vi "prop_plot_main.vi"() -> ()   [LabVIEW 2020, in "3DPC_SurfacePlot.xctl"]
uses:
  <vilib>/Native 3D Graph/xcontrol/3DPC_SurfacePlot.xctl
  <vilib>/Native 3D Graph/typedefs/prop_plot_all_array.ctl
  <vilib>/Native 3D Graph/typedefs/prop_plot_all.ctl
  <vilib>/Native 3D Graph/typedefs/prop_plot_projection.ctl
  <vilib>/Native 3D Graph/typedefs/prop_plot_surface.ctl
  <vilib>/Native 3D Graph/typedefs/prop_plot_contour.ctl
  <vilib>/Native 3D Graph/typedefs/prop_plot_normal.ctl
  <vilib>/Native 3D Graph/typedefs/prop_plot_point_line.ctl
  <vilib>/Native 3D Graph/typedefs/range_cluster.ctl
  <vilib>/Native 3D Graph/typedefs/min_max.ctl
  <vilib>/Utility/miscctls.llb/LVPointTypeDef.ctl
  <vilib>/Utility/miscctls.llb/LVPositionTypeDef.ctl
  <vilib>/event_ctls.llb/eventvkey.ctl
panel:
  in  "add new":string="[add new]"
  in  "Min Max":T1
  in  "done":refnum<user-event>
  in  "quit":refnum<user-event>
  out "Plot Properties Out":T3
  in  "Plot Properties In":T3
  in  "Delete Plot":bool
  in  "Add Plot":bool
  in  "Plots":i32(listbox)
  in  "Tab Plot Prop":T10(tab)
  in  "Color Map Mode":u16(ring) items=["Absolute", "Relative"]
  in  "Autoscale":bool
  in  "Coordinate System":u16(ring) items=["Cartesian", "Cylindrical", "Spherical"]
  in  "Surface Opacity":dbl=1.0 caption="Opacity"
  in  "Surface Shading":bool
  in  "Surface Draw":bool
  in  "Color Ramp":dbl(ramp) caption="Color Map"
  in  "Point Size":sgl=1.0
  in  "PL Color":u32(colorbox) caption="Color"
  in  "PL Antialiasing":bool
  in  "Points/Lines":u16(ring) items=["None", "Points", "Lines", "Both"]
  in  "Point Style":u16(ring) items=["Point", "EmptySquare", "Asterisk", "Diamond", "EmptyCircle", "Circle", "X"]
  in  "Line Style":u16(ring) items=["Solid", "Dash", "Dot", "Dash Dot"]
  in  "Line Width":sgl=1.0
  in  "Level List":i32(listbox)
  in  "Mode":u16(ring) items=["Levels", "Intervals", "Level List"]
  in  "Anchored Num":dbl
  in  "Anchored at":bool
  in  "Levels":sgl
  in  "Contour Direction":u16(ring) caption="Axis" items=["X", "Y", "Z"]
  in  "Contour Width":dbl=1.0 caption="Width"
  in  "Contour Color":u32(colorbox) caption="Color"
  in  "Contour Antialiasing":bool
  in  "Contour Draw":bool
  in  "Contour Line Style":u16(ring) caption="Line Style" items=["Solid", "Dash", "Dot", "Dash Dot"]
  in  "Interval":sgl
  in  "Normal Color":u32(colorbox) caption="Color"
  in  "Normal Length":sgl=0.1 caption="Length"
  in  "Normal Width":sgl=3.0 caption="Width"
  in  "Normal Draw":bool
  in  "Normal Antialiasing":bool
  in  "Projection Draw XY":bool
  in  "Projection Draw YZ":bool
  in  "Projection Draw XZ":bool
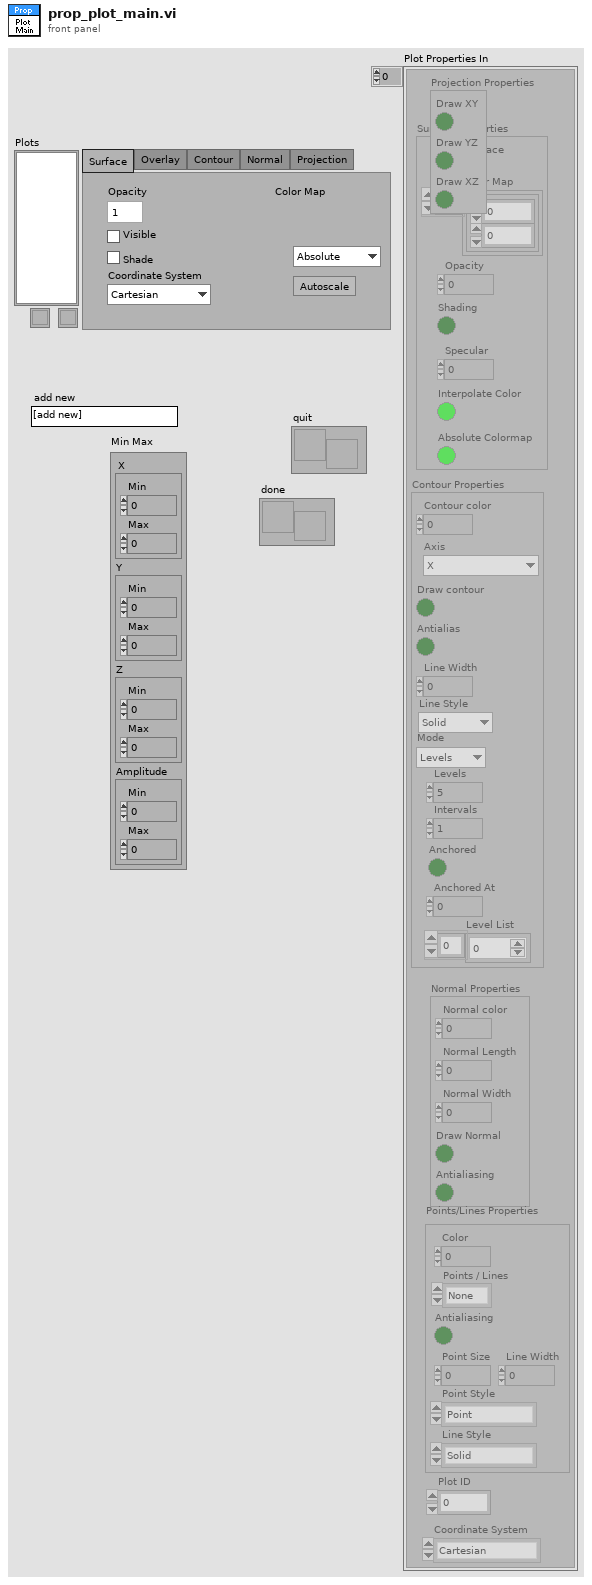
[diagram p1: front panel]
types:
  T1 = typedef "3DPC_SurfacePlot.xctl/range_cluster.ctl" = cluster{"X":T2, "Y":T2, "Z":T2, "Amplitude":T2}
  T2 = typedef "3DPC_SurfacePlot.xctl/min_max.ctl" = cluster{"Min":sgl, "Max":sgl}
  T3 = typedef "3DPC_SurfacePlot.xctl/prop_plot_all_array.ctl" = T4[]
  T4 = typedef "3DPC_SurfacePlot.xctl/prop_plot_all.ctl" = cluster{"Projection Properties":T5, "Surface Properties":T6, "Contour Properties":T7, "Normal Properties":T8, "Points/Lines Properties":T9, "Plot ID":i32, "Coordinate System":enum16{"Cartesian", "Cylindrical", "Spherical"}}
  T5 = typedef "3DPC_SurfacePlot.xctl/prop_plot_projection.ctl" = cluster{"Draw XY":bool, "Draw YZ":bool, "Draw XZ":bool}
  T6 = typedef "3DPC_SurfacePlot.xctl/prop_plot_surface.ctl" = cluster{"Draw surface":bool, "Opacity":dbl, "Shading":bool, "Specular":i32, "Color Map":cluster{dbl, u32}[], "Interpolate Color":bool, "Absolute Colormap":bool}
  T7 = typedef "3DPC_SurfacePlot.xctl/prop_plot_contour.ctl" = cluster{"Contour color":u32, "Axis":enum16{"X", "Y", "Z"}, "Draw contour":bool, "Antialias":bool, "Line Width":sgl, "Contour Line Style":enum16{"Solid", "Dash", "Dot", "Dash Dot"}, "Mode":enum16{"Levels", "Intervals", "Level List"}, "Levels":sgl, "Intervals":sgl, "Anchored At":sgl, "Anchored":bool, "Level List":dbl[]}
  T8 = typedef "3DPC_SurfacePlot.xctl/prop_plot_normal.ctl" = cluster{"Normal color":u32, "Normal Length":sgl, "Normal Width":sgl, "Draw Normal":bool, "Antialiasing":bool}
  T9 = typedef "3DPC_SurfacePlot.xctl/prop_plot_point_line.ctl" = cluster{"Color":u32, "Antialiasing":bool, "Point Size":sgl, "Points / Lines":enum16{"None", "Points", "Lines", "Both"}, "Point Style":enum16{"Point", "EmptySquare", "Asterisk", "Diamond", "EmptyCircle", "Circle", "X"}, "Line Style":enum16{"Solid", "Dash", "Dot", "Dash Dot"}, "Line Width":sgl}
  T10 = enum32{"Surface", "Overlay", "Contour", "Normal", "Projection"}
  T11 = typedef "LVPointTypeDef.ctl" = cluster{"Horizontal":i16, "Vertical":i16}
  T12 = typedef "LVPositionTypeDef.ctl" = cluster{"Left":i32, "Top":i32}
  T13 = typedef "eventvkey.ctl" = enum16{"ASCII", "Enter", "Return", "Shift", "Ctrl", "Alt", "Cmd", "Opt", "Caps", "NumLock", "Clear", "Break", "Up", "Down", "Left", "Right", "Insert", "Delete", "Home", "End", "PageUp", "PageDown", "Escape", "Help", "Pause", "ScrollLock", "F1", "F2", "F3", "F4", "F5", "F6", "F7", "F8", "F9", "F10", "F11", "F12", "F13", "F14", "F15", "F16", "F17", "F18", "F19", "F20", "F21", "F22", "F23", "F24", "Play", "VolumeUp", "VolumeDown", "Mute", "Two Byte Char"}
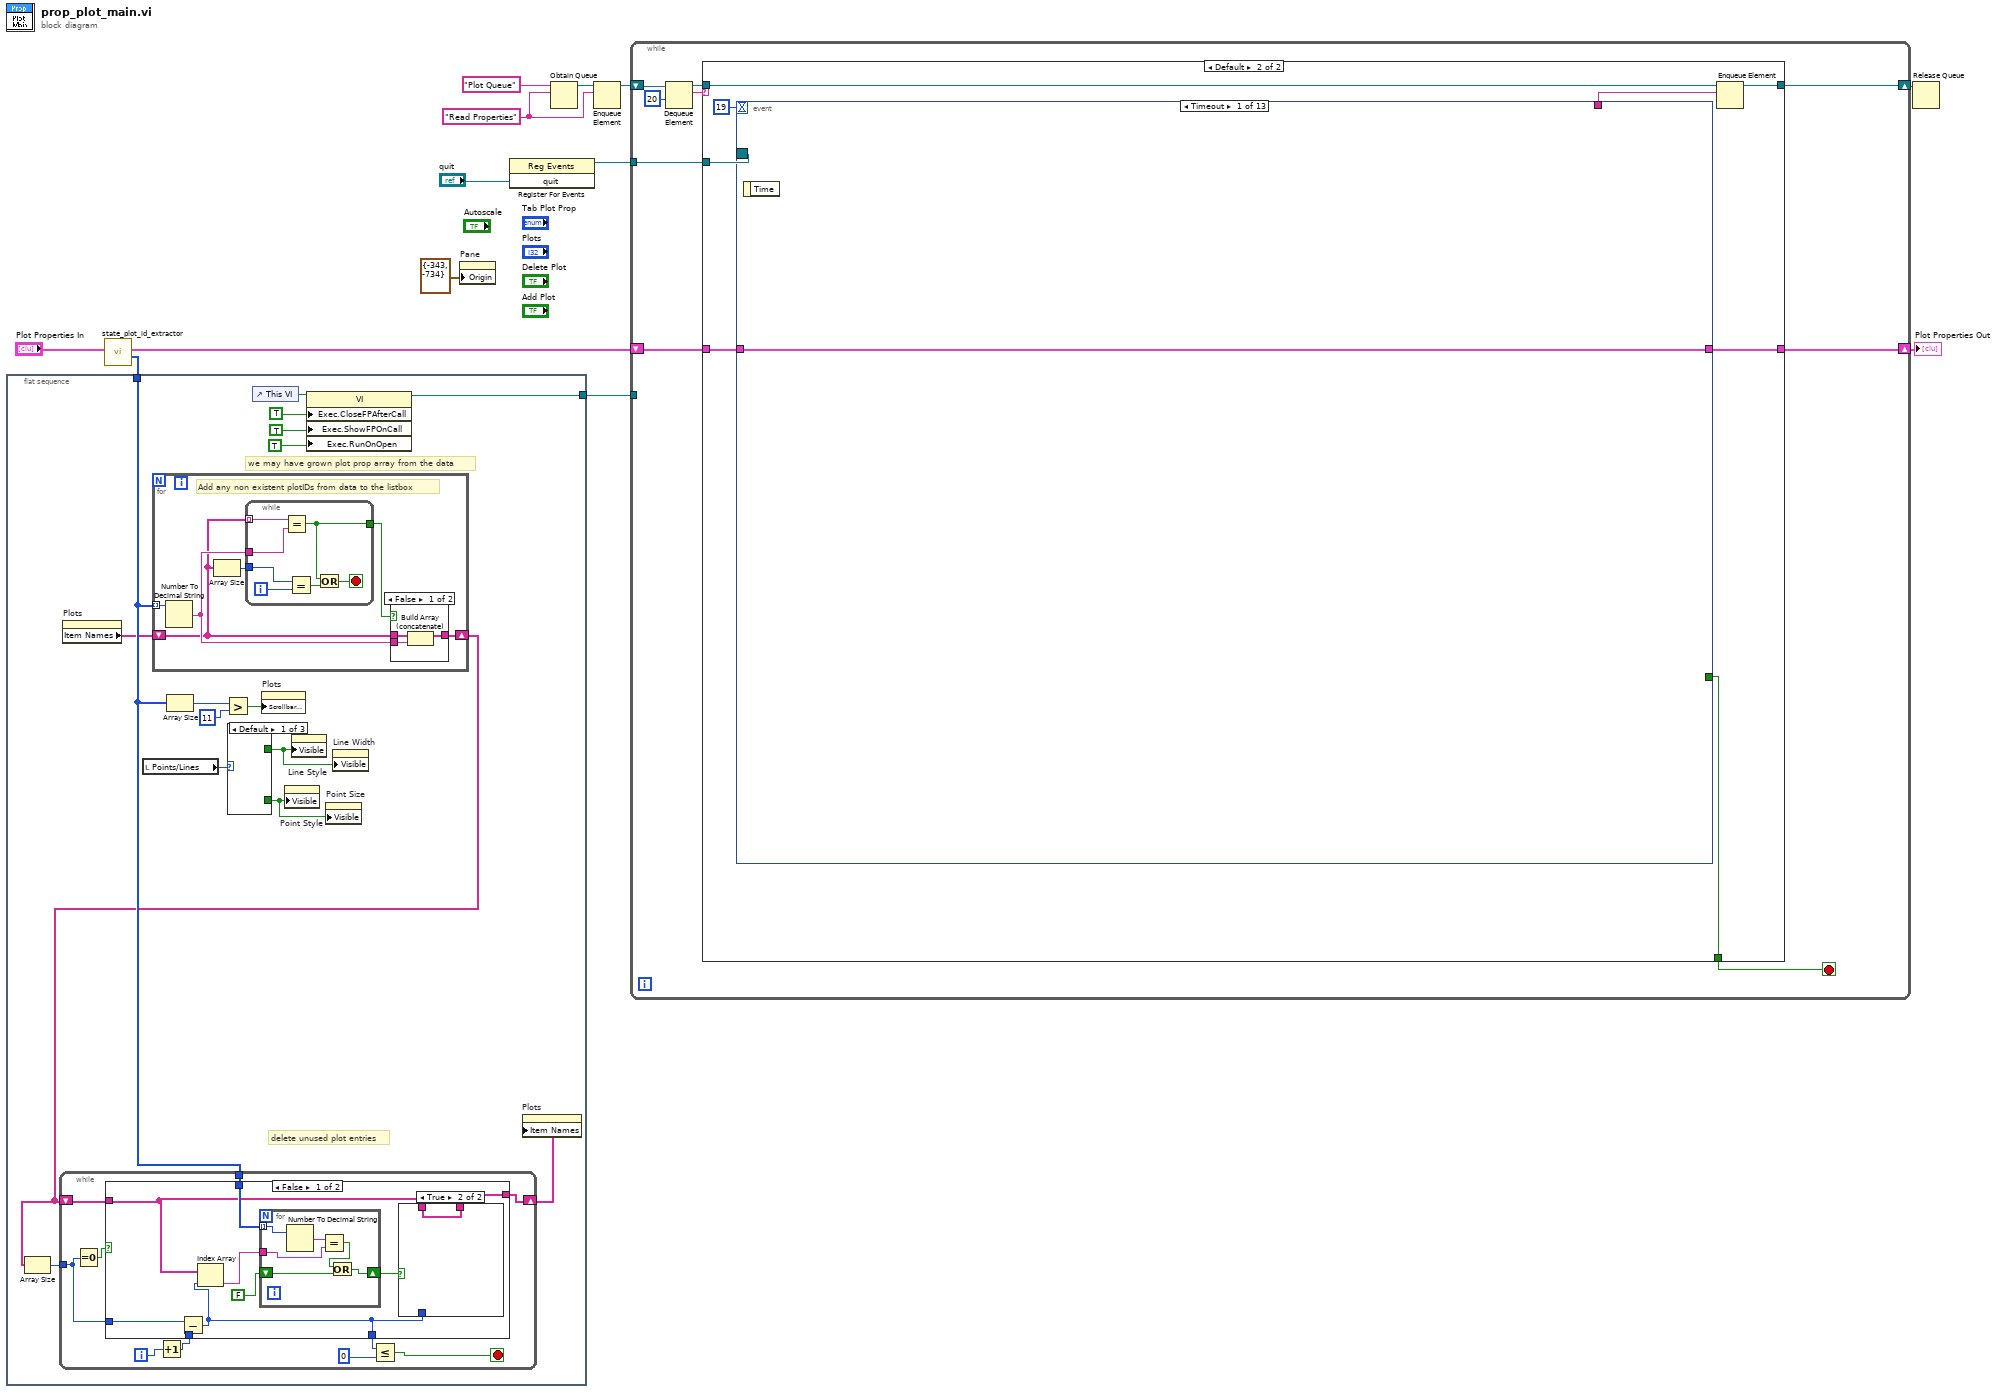
[diagram p0: block diagram]
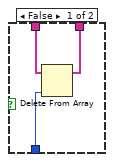
[diagram p2: hidden frame]
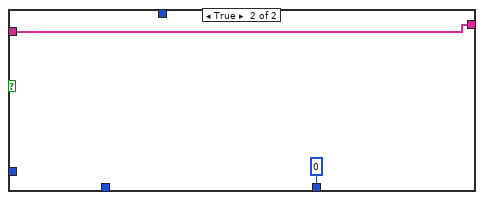
[diagram p3: hidden frame]
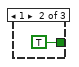
[diagram p4: hidden frame]
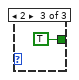
[diagram p5: hidden frame]
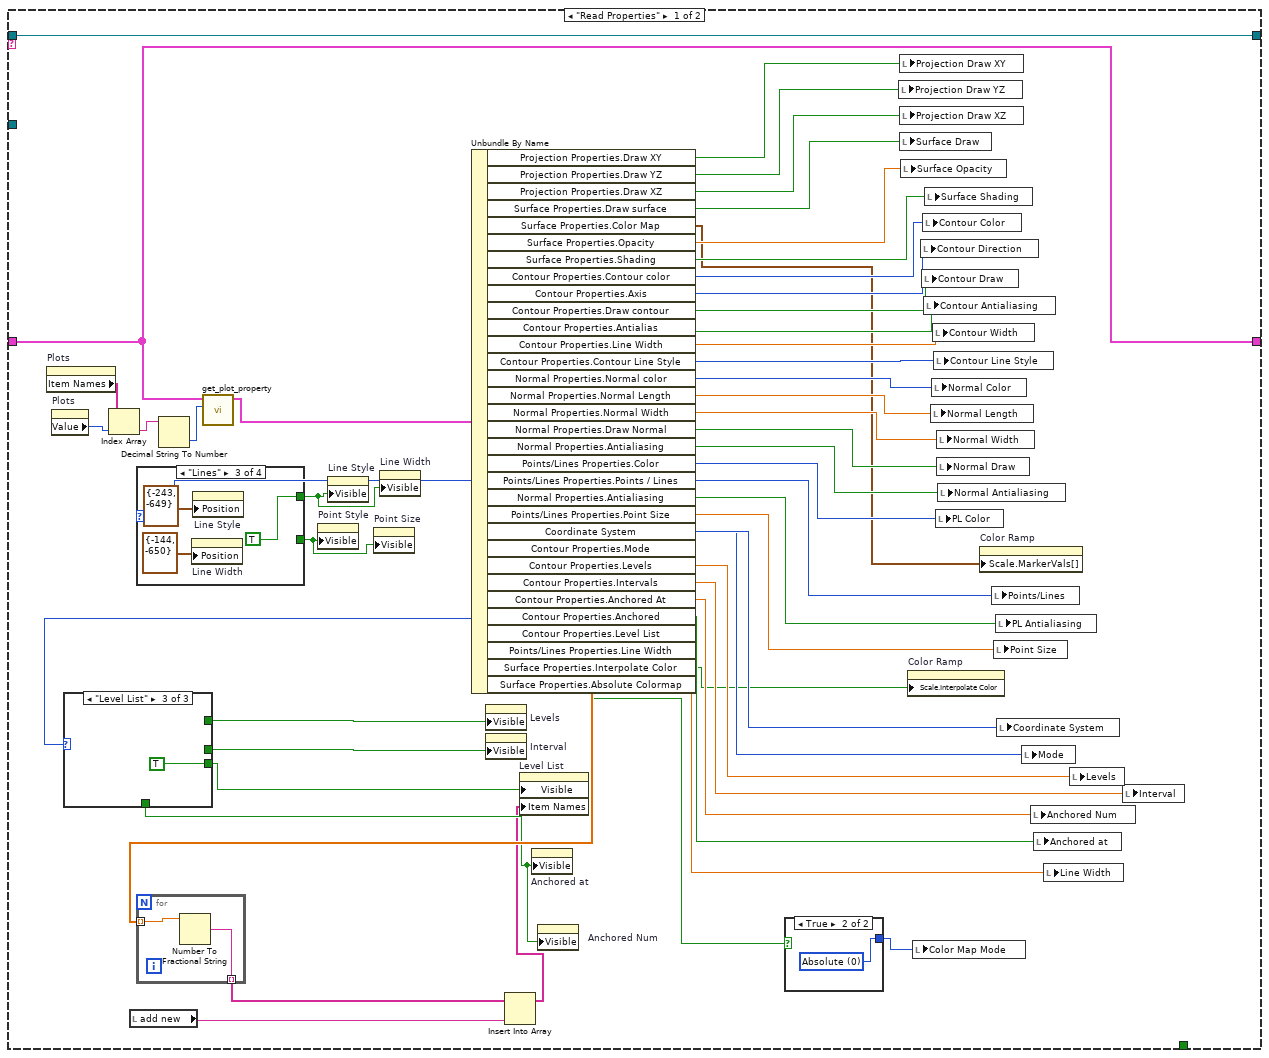
[diagram p7: hidden frame]
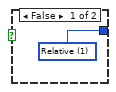
[diagram p8: hidden frame]
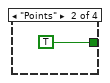
[diagram p10: hidden frame]
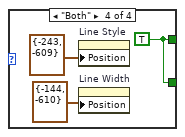
[diagram p11: hidden frame]
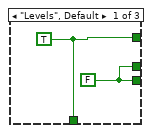
[diagram p12: hidden frame]
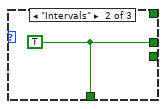
[diagram p13: hidden frame]
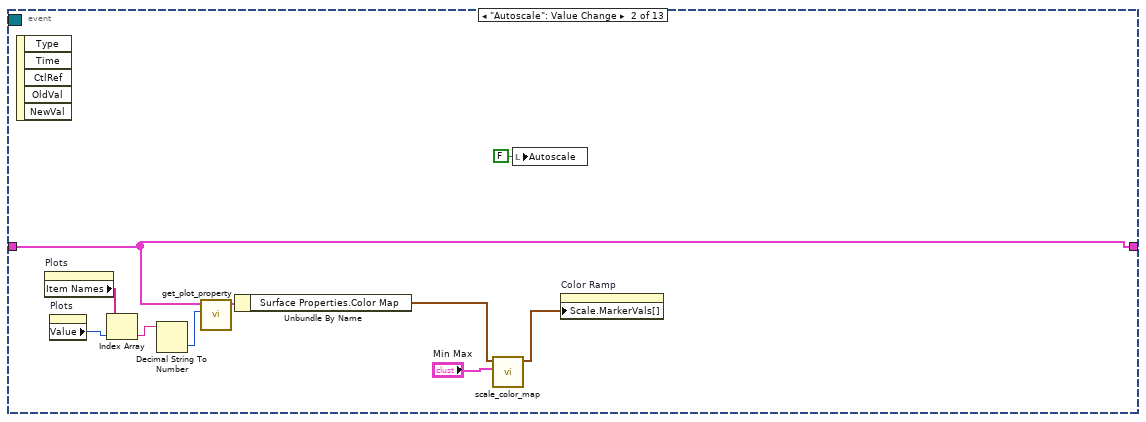
[diagram p14: hidden frame]
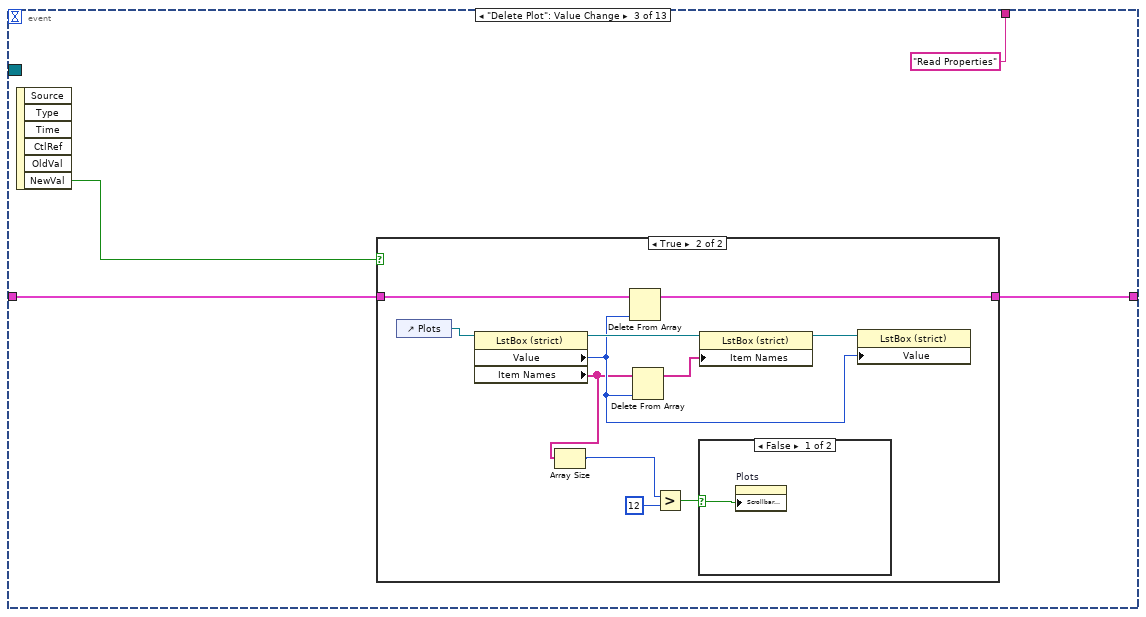
[diagram p15: hidden frame]
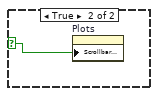
[diagram p17: hidden frame]
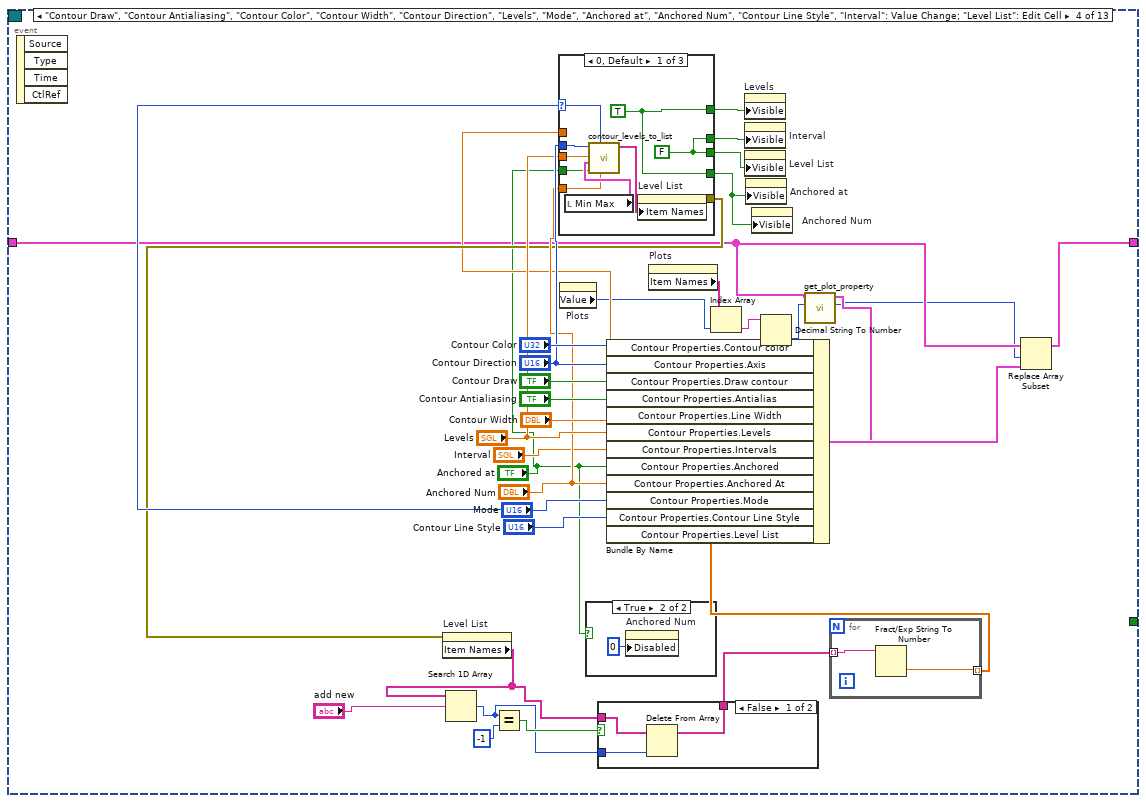
[diagram p18: hidden frame]
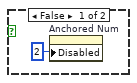
[diagram p19: hidden frame]
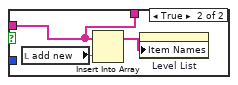
[diagram p20: hidden frame]
diagram:
  w11 = "Read Properties"
  n1 = flat-sequence {
    tunnel: [w29] -> w7
    tunnel: w4 -> [w28]
    frame #0 {
      # "delete unused plot entries"
      # "we may have grown plot prop array from the data"
      n2 = property on="Plots" class="LstBox (strict)"() -> ("Item Names"=w14:string[])  [unwired: 2 in, 2 out]
      n3 = local read "Points/Lines"() -> (w21:u16)
      n4 = for {
        tunnel: w28 -> [w66] mode=indexing
        shift-right: [w64] -> w16
        shift-left: w14 -> [w63]
        # "Add any non existent plotIDs from data to the listbox"
        n5 = Number To Decimal String(number=w66) -> (decimal integer string=w65:string)  [unwired: 1 out]
        n6 = Array Size(array=w63) -> (size(s)=w68:i32)
        n7 = while {
          tunnel: w63 -> [w79] mode=indexing
          tunnel: w68 -> [w78]
          tunnel: [w74] -> w67
          tunnel: w65 -> [w73]
          i -> [w77]
          stop <- w75 stop-if-true
          n8 = Equal?(x=w79, y=w73) -> (x = y?=w74:bool)
          n9 = Equal?(x=w78, y=w77) -> (x = y?=w76:bool)
          n10 = Or(x=w74, y=w76) -> (x .or. y?=w75:bool)
        }
        n11 = case shown="False" w67 {
          tunnel: w65 -> [w71 _]
          tunnel: [w70 w72] -> w64
          tunnel: w63 -> [w69 w72]
          frame False {
            n12 = Build Array (concatenate)(w69, w71) -> (w70:string[])
          }
          frame True {
          }
        }
      }
      n13 = Array Size(array=w16) -> (size(s)=w15:i32)
      n14 = while {
        tunnel: w28 -> [w37]
        shift-right: [w36] -> w17
        shift-left: w16 -> [w35]
        tunnel: w15 -> [w31]
        i -> [w38]
        stop <- w32 stop-if-true
        n15 = Equal To 0?(x=w31) -> (x = 0?=w30:bool)
        n16 = Increment(x=w38) -> (x+1=w39:i32)
        n17 = case shown="False" w30 {
          tunnel: w39 -> [w48 _]
          tunnel: w37 -> [w47 _]
          tunnel: [w44 w60] -> w36
          tunnel: w35 -> [w42 w60]
          tunnel: [w41 0] -> w34
          tunnel: w31 -> [w40 _]
          frame False {
            n18 = Subtract(x=w40, y=w48) -> (x-y=w41:i32)
            n19 = Index Array(array=w42, index=w41) -> (element=w46:string)
            n20 = for {
              tunnel: w47 -> [w58] mode=indexing
              tunnel: w46 -> [w56]
              shift-right: [w53] -> w43
              shift-left: FALSE -> [w55]
              n21 = Number To Decimal String(number=w58) -> (decimal integer string=w57:string)  [unwired: 1 out]
              n22 = Equal?(x=w57, y=w56) -> (x = y?=w54:bool)
              n23 = Or(x=w54, y=w55) -> (x .or. y?=w53:bool)
            }
            n24 = case shown="True" w43 {
              tunnel: w42 -> [w50 w52]
              tunnel: w41 -> [w51 _]
              tunnel: [w49 w52] -> w44
              frame False {
                n25 = Delete From Array(array=w50, index=w51) -> (array with subset deleted=w49:string[])  [unwired: 1 in, 1 out]
              }
              frame True {
              }
            }
          }
          frame True {
          }
        }
        n26 = Less Or Equal?(x=w34, y=0) -> (x <= y?=w32:bool)
      }
      n27 = Array Size(array=w28) -> (size(s)=w20:i32)
      n28 = Greater?(x=w20, y=11) -> (0:w18:bool)
      n29 = case shown="Default" w21 {
        tunnel: [_ TRUE ("Visible") _] -> w23
        tunnel: [_ _ TRUE ("Visible")] -> w22
        frame Default {
        }
        frame 1 {
        }
        frame 2 {
        }
      }
      n30 = control-ref of="This VI"() -> (w27:refnum<vi>)
      n31 = property on="Plots" class="LstBox (strict)"("Scrollbar Visible"=w18) -> ()  [unwired: 2 in, 2 out]
      n32 = property on="Point Style" class="Ring (strict)"("Visible"=w23) -> ()  [unwired: 2 in, 2 out]
      n33 = property on="Line Style" class="Ring (strict)"("Visible"=w22) -> ()  [unwired: 2 in, 2 out]
      n34 = property class="VI"(reference=w27, "Exec.CloseFPAfterCall"=TRUE ("Execution:Close After Call"), "Exec.ShowFPOnCall"=TRUE ("Execution:Show Front Panel On Call"), "Exec.RunOnOpen"=TRUE ("Execution:Run When Opened")) -> (reference out=w29:refnum<vi>)  [unwired: 1 in, 1 out]
      n35 = property on="Point Size" class="DigNum (strict)"("Visible"=w23) -> ()  [unwired: 2 in, 2 out]
      n36 = property on="Line Width" class="DigNum (strict)"("Visible"=w22) -> ()  [unwired: 2 in, 2 out]
      n37 = property on="Plots" class="LstBox (strict)"("Item Names"=w17) -> ()  [unwired: 2 in, 2 out]
    }
  }
  n38 = call <vilib>:"state_plot_id_extractor.vi"("Plot Properties Array In"="Plot Properties In") -> ("Plot IDs"=w4:i32[], "Plot Properties Array Out"=w5:T3)  [unwired: 9 out]
  n39 = property on="Pane" class="Pane"("Origin"=T11 {"Horizontal"=-343, "Vertical"=-734} ("Point")) -> ()  [unwired: 2 in, 2 out]
  n40 = register-events("quit") -> (reference out=w2:refnum<event-registration>)  [unwired: 2 in, 1 out]
  n41 = Obtain Queue(name (unnamed)="Plot Queue", element data type=w11) -> (queue out=w12:refnum<queue>)  [unwired: 3 in, 2 out]
  n42 = Enqueue Element(queue=w12, element=w11) -> (queue out=w10:refnum<queue>)  [unwired: 1 in, 3 out]
  n43 = while {
    shift-right: [w87] -> w9
    shift-left: w5 -> [w88]
    shift-right: [w82] -> w8
    shift-left: w10 -> [w85]
    tunnel: w7 -> [_]
    tunnel: w2 -> [w81]
    stop <- w80 stop-if-true
    n44 = Dequeue Element(queue=w85, timeout in ms (-1)=20) -> (queue out=w83:refnum<queue>, element=w84:string)  [unwired: 1 in, 2 out]
    n45 = case shown="Default" w84 {
      tunnel: w88 -> [w98 w157]
      tunnel: [w98 w156] -> w87
      tunnel: w83 -> [w137 w160]
      tunnel: [w137 w159] -> w82
      tunnel: w81 -> [_ w154]
      tunnel: [_ w153] -> w80
      frame "Read Properties" {
        n46 = property on="Plots" class="LstBox (strict)"() -> ("Item Names"=w96:string[])  [unwired: 2 in, 2 out]
        n47 = property on="Plots" class="LstBox (strict)"() -> ("Value"=w95:i32)  [unwired: 2 in, 2 out]
        n48 = Index Array(array=w96, index=w95) -> (element=w94:string)
        n49 = local read "add new"() -> (w99:string)
        n50 = Decimal String To Number(string=w94) -> (number=w93:i32)  [unwired: 3 out]
        n51 = call <vilib>:"get_plot_property.vi"("Plot ID"=w93, "Plot Properties Array"=w98) -> ("element"=w97:T4)  [unwired: 1 in, 8 out]
        n52 = Unbundle By Name(w97) -> ("Projection Properties.Draw XY"=w136:bool, "Projection Properties.Draw YZ"=w135:bool, "Projection Properties.Draw XZ"=w134:bool, "Surface Properties.Draw surface"=w133:bool, "Surface Properties.Color Map"=w92:cluster{dbl, u32}[], "Surface Properties.Opacity"=w132:dbl, "Surface Properties.Shading"=w131:bool, "Contour Properties.Contour color"=w130:u32, "Contour Properties.Axis"=w129:enum16{"X", "Y", "Z"}, "Contour Properties.Draw contour"=w128:bool, "Contour Properties.Antialias"=w127:bool, "Contour Properties.Line Width"=w126:sgl, "Contour Properties.Contour Line Style"=w116:enum16{"Solid", "Dash", "Dot", "Dash Dot"}, "Normal Properties.Normal color"=w125:u32, "Normal Properties.Normal Length"=w124:sgl, "Normal Properties.Normal Width"=w123:sgl, "Normal Properties.Draw Normal"=w122:bool, "Normal Properties.Antialiasing"=w121:bool, "Points/Lines Properties.Color"=w120:u32, "Points/Lines Properties.Points / Lines"=w101:enum16{"None", "Points", "Lines", "Both"}, "Normal Properties.Antialiasing"=w119:bool, "Points/Lines Properties.Point Size"=w118:sgl, "Coordinate System"=w117:enum16{"Cartesian", "Cylindrical", "Spherical"}, "Contour Properties.Mode"=w113:enum16{"Levels", "Intervals", "Level List"}, "Contour Properties.Levels"=w111:sgl, "Contour Properties.Intervals"=w110:sgl, "Contour Properties.Anchored At"=w109:sgl, "Contour Properties.Anchored"=w108:bool, "Contour Properties.Level List"=w107:dbl[], "Points/Lines Properties.Line Width"=w100:sgl, "Surface Properties.Interpolate Color"=w91:bool, "Surface Properties.Absolute Colormap"=w90:bool)
        n53 = case shown="\"Level List\"" w113 {
          tunnel: [w149 _ _] -> w115
          tunnel: [w150 w151 _] -> w114
          tunnel: [w150 _ TRUE ("Visible")] -> w112
          tunnel: [w149 w151 _] -> w106
          frame "Levels", Default {
            w150 = FALSE ("Visible")
            w149 = TRUE ("Visible")
          }
          frame "Intervals" {
            w151 = TRUE ("Visible")
          }
          frame "Level List" {
          }
        }
        n54 = case shown="\"Lines\"" w101 {
          tunnel: [_ TRUE ("Visible") _ w144] -> w102
          tunnel: [_ _ TRUE ("Visible") w144] -> w103
          frame "None", Default {
          }
          frame "Points" {
          }
          frame "Lines" {
            n55 = property on="Line Width" class="DigNum (strict)"("Position"=T12 {"Left"=-144, "Top"=-650} ("Position 3")) -> ()  [unwired: 2 in, 2 out]
            n56 = property on="Line Style" class="Ring (strict)"("Position"=T12 {"Left"=-243, "Top"=-649} ("Position 2")) -> ()  [unwired: 2 in, 2 out]
          }
          frame "Both" {
            w144 = TRUE ("Visible")
            n57 = property on="Line Style" class="Ring (strict)"("Position"=T12 {"Left"=-243, "Top"=-609} ("Position 4")) -> ()  [unwired: 2 in, 2 out]
            n58 = property on="Line Width" class="DigNum (strict)"("Position"=T12 {"Left"=-144, "Top"=-610} ("Position 5")) -> ()  [unwired: 2 in, 2 out]
          }
        }
        n59 = for {
          tunnel: w107 -> [w148] mode=indexing
          tunnel: [w147] -> w105 mode=indexing
          n60 = Number To Fractional String(number=w148) -> (F-format string=w147:string)  [unwired: 3 out]
        }
        n61 = property on="Point Style" class="Ring (strict)"("Visible"=w102) -> ()  [unwired: 2 in, 2 out]
        n62 = property on="Line Style" class="Ring (strict)"("Visible"=w103) -> ()  [unwired: 2 in, 2 out]
        n63 = property on="Point Size" class="DigNum (strict)"("Visible"=w102) -> ()  [unwired: 2 in, 2 out]
        n64 = property on="Line Width" class="DigNum (strict)"("Visible"=w103) -> ()  [unwired: 2 in, 2 out]
        n65 = property on="Levels" class="DigNum (strict)"("Visible"=w115) -> ()  [unwired: 2 in, 2 out]
        n66 = property on="Interval" class="DigNum (strict)"("Visible"=w114) -> ()  [unwired: 2 in, 2 out]
        n67 = Insert Into Array(array=w105, new element=w99) -> (w104:string[])  [unwired: 1 in]
        n68 = property on="Level List" class="LstBox (strict)"("Visible"=w112, "Item Names"=w104) -> ()  [unwired: 2 in, 2 out]
        n69 = property on="Anchored at" class="Bool (strict)"("Visible"=w106) -> ()  [unwired: 2 in, 2 out]
        n70 = property on="Anchored Num" class="DigNum (strict)"("Visible"=w106) -> ()  [unwired: 2 in, 2 out]
        n71 = case shown="True" w90 {
          tunnel: [w138 w139] -> w89
          frame False {
            w138 = u16 1 items=["Absolute", "Relative"] ("Color Map Mode")
          }
          frame True {
            w139 = u16 0 items=["Absolute", "Relative"] ("Color Map Mode")
          }
        }
        n72 = local write "Projection Draw YZ"(w135) -> ()
        n73 = local write "Projection Draw XY"(w136) -> ()
        n74 = local write "Projection Draw XZ"(w134) -> ()
        n75 = local write "Surface Draw"(w133) -> ()
        n76 = local write "Surface Opacity"(w132) -> ()
        n77 = property on="Color Ramp" class="ColRmp (strict)"("Scale.Interpolate Color"=w91) -> ()  [unwired: 2 in, 2 out]
        n78 = local write "Color Map Mode"(w89) -> ()
        n79 = local write "Contour Direction"(w129) -> ()
        n80 = local write "Contour Draw"(w128) -> ()
        n81 = local write "Contour Color"(w130) -> ()
        n82 = local write "Contour Antialiasing"(w127) -> ()
        n83 = local write "Surface Shading"(w131) -> ()
        n84 = local write "Normal Length"(w124) -> ()
        n85 = local write "Normal Color"(w125) -> ()
        n86 = local write "Contour Width"(w126) -> ()
        n87 = local write "Contour Line Style"(w116) -> ()
        n88 = local write "PL Color"(w120) -> ()
        n89 = local write "Normal Width"(w123) -> ()
        n90 = local write "Normal Draw"(w122) -> ()
        n91 = local write "Normal Antialiasing"(w121) -> ()
        n92 = property on="Color Ramp" class="ColRmp (strict)"("Scale.MarkerVals[]"=w92) -> ()  [unwired: 2 in, 2 out]
        n93 = local write "Points/Lines"(w101) -> ()
        n94 = local write "Point Size"(w118) -> ()
        n95 = local write "PL Antialiasing"(w119) -> ()
        n96 = local write "Coordinate System"(w117) -> ()
        n97 = local write "Mode"(w113) -> ()
        n98 = local write "Anchored Num"(w109) -> ()
        n99 = local write "Anchored at"(w108) -> ()
        n100 = local write "Line Width"(w100) -> ()
        n101 = local write "Levels"(w111) -> ()
        n102 = local write "Interval"(w110) -> ()
      }
      frame Default {
        n103 = event shown="[0] Timeout" {
          selector: w154 -> [_ _ _ _ _ _ _ _ _ _ _ _ _]
          dyn-events: _ -> [_ _ _ _ _ _ _ _ _ _ _ _ _]
          timeout: 19 -> [_ _ _ _ _ _ _ _ _ _ _ _ _]
          tunnel: [_ _ "Read Properties" ("element") _ _ _ "Read Properties" ("element") _ _ "Read Properties" ("element") _ _ _] -> w158
          tunnel: w157 -> [w161 w166 w174 w194 w252 w289 w302 w312 w322 w339 w357 w368 w401]
          tunnel: [w161 w166 w173 w220 w251 w298 w308 w319 w329 w338 w362 w383 w415] -> w156
          tunnel: [_ _ _ _ _ _ _ _ TRUE _ _ _ _] -> w153
          event Timeout {
            n104 = event-data() -> ()  [unwired: 2 out]
          }
          event "Autoscale": Value Change {
            n105 = event-data() -> ()  [unwired: 6 out]
            n106 = property on="Plots" class="LstBox (strict)"() -> ("Item Names"=w171:string[])  [unwired: 2 in, 2 out]
            n107 = property on="Plots" class="LstBox (strict)"() -> ("Value"=w170:i32)  [unwired: 2 in, 2 out]
            n108 = Index Array(array=w171, index=w170) -> (element=w169:string)
            n109 = Decimal String To Number(string=w169) -> (number=w168:i32)  [unwired: 3 out]
            n110 = call <vilib>:"get_plot_property.vi"("Plot ID"=w168, "Plot Properties Array"=w166) -> ("element"=w167:T4)  [unwired: 1 in, 8 out]
            n111 = Unbundle By Name(w167) -> ("Surface Properties.Color Map"=w164:cluster{dbl, u32}[])
            n112 = call <vilib>:"scale_color_map.vi"("Min Max"="Min Max", "Color Map In"=w164) -> ("Color Map Out"=w163:cluster{dbl, u32}[])  [unwired: 9 out]
            n113 = local write "Autoscale"(FALSE ("Autoscale")) -> ()
            n114 = property on="Color Ramp" class="ColRmp (strict)"("Scale.MarkerVals[]"=w163) -> ()  [unwired: 2 in, 2 out]
          }
          event "Delete Plot": Value Change {
            n115 = event-data() -> ("NewVal"=w175:bool)  [unwired: 6 out]
            n116 = case shown="True" w175 {
              tunnel: w174 -> [w176 w187]
              tunnel: [w176 w186] -> w173
              frame False {
              }
              frame True {
                n117 = control-ref of="Plots"() -> (w184:refnum<vi>)
                n118 = property on="Property Node" class="LstBox (strict)"(reference=w184) -> (reference out=w183:refnum<vi>, "Value"=w181:i32, "Item Names"=w178:string[])  [unwired: 1 in, 1 out]
                n119 = Array Size(array=w178) -> (size(s)=w177:i32)
                n120 = Delete From Array(array=w187, index=w181) -> (array with subset deleted=w186:T3)  [unwired: 1 in, 1 out]
                n121 = Delete From Array(array=w178, index=w181) -> (array with subset deleted=w185:string[])  [unwired: 1 in, 1 out]
                n122 = Greater?(x=w177, y=12) -> (0:w180:bool)
                n123 = case shown="False" w180 {
                  selector: w180 -> [w188 w189]
                  frame False {
                    n124 = property on="Plots" class="LstBox (strict)"("Scrollbar Visible"=w188) -> ()  [unwired: 2 in, 2 out]
                  }
                  frame True {
                    n125 = property on="Plots" class="LstBox (strict)"("Scrollbar Visible"=w189) -> ()  [unwired: 2 in, 2 out]
                  }
                }
                n126 = property on="Property Node" class="LstBox (strict)"(reference=w183, "Item Names"=w185) -> (reference out=w182:refnum<vi>)  [unwired: 1 in, 1 out]
                n127 = property class="LstBox (strict)"(reference=w182, "Value"=w181) -> ()  [unwired: 1 in, 2 out]
              }
            }
          }
          event "Contour Draw", "Contour Antialiasing", "Contour Color", "Contour Width", "Contour Direction", "Levels", "Mode", "Anchored at", "Anchored Num", "Contour Line Style", "Interval": Value Change; "Level List": Edit Cell {
            n128 = event-data() -> ()  [unwired: 5 out]
            n129 = case shown="0, Default" "Mode" {
              selector: "Mode" -> [w230 w242 _]
              tunnel: [w238 _ _] -> w212
              tunnel: [w239 w247 _] -> w211
              tunnel: [w239 _ TRUE ("Visible")] -> w210
              tunnel: [w238 w247 _] -> w209
              tunnel: "Contour Direction" -> [w237 w243 _]
              tunnel: "Levels" -> [w231 _ _]
              tunnel: "Anchored at" -> [w235 w244 _]
              tunnel: "Anchored Num" -> [w234 w241 _]
              tunnel: [w232 _ _] -> w205
              tunnel: "Interval" -> [_ w240 _]
              frame 0, Default {
                w239 = FALSE ("Visible")
                w238 = TRUE ("Visible")
                n130 = local read "Min Max"() -> (w236:T1)
                n131 = call <vilib>:"contour_levels_to_list.vi"("Anchored Num"=w234, "Mode"=w230, "Anchored at"=w235, "Min Max"=w236, "Levels/Int"=w231, "Dimension"=w237) -> ("Item Names"=w233:string[])  [unwired: 5 out]
                n132 = property on="Level List" class="LstBox (strict)"("Item Names"=w233) -> (error out=w232:errorcluster)  [unwired: 2 in, 1 out]
              }
              frame 1 {
                w247 = TRUE ("Visible")
                n133 = local read "Min Max"() -> (w245:T1)
                n134 = call <vilib>:"contour_levels_to_list.vi"("Anchored Num"=w241, "Mode"=w242, "Anchored at"=w244, "Min Max"=w245, "Levels/Int"=w240, "Dimension"=w243) -> ("Item Names"=w246:string[])  [unwired: 5 out]
                n135 = property on="Level List" class="LstBox (strict)"("Item Names"=w246) -> ()  [unwired: 2 in, 2 out]
              }
              frame 2 {
              }
            }
            n136 = property on="Level List" class="LstBox (strict)"(error in=w205) -> ("Item Names"=w201:string[])  [unwired: 1 in, 2 out]
            n137 = Search 1D Array(1D array=w201, element="add new") -> (index of element=w200:i32)  [unwired: 1 out]
            n138 = Equal?(x=w200, y=-1) -> (x = y?=w202:bool)
            n139 = property on="Plots" class="LstBox (strict)"() -> ("Value"=w192:i32)  [unwired: 2 in, 2 out]
            n140 = case shown="True" "Anchored at" {
              frame False {
                n141 = property on="Anchored Num" class="DigNum (strict)"("Disabled"=u8 2) -> ()  [unwired: 2 in, 2 out]
              }
              frame True {
                n142 = property on="Anchored Num" class="DigNum (strict)"("Disabled"=u8 0) -> ()  [unwired: 2 in, 2 out]
              }
            }
            n143 = case shown="False" w202 {
              tunnel: w201 -> [w224 w229]
              tunnel: [w225 w229] -> w199
              tunnel: w200 -> [w226 _]
              frame False {
                n144 = Delete From Array(array=w224, index=w226) -> (array with subset deleted=w225:string[])  [unwired: 1 in, 1 out]
              }
              frame True {
                n145 = local read "add new"() -> (w227:string)
                n146 = Insert Into Array(array=w229, new element=w227) -> (w228:string[])  [unwired: 1 in]
                n147 = property on="Level List" class="LstBox (strict)"("Item Names"=w228) -> ()  [unwired: 2 in, 2 out]
              }
            }
            n148 = property on="Plots" class="LstBox (strict)"() -> ("Item Names"=w196:string[])  [unwired: 2 in, 2 out]
            n149 = Index Array(array=w196, index=w192) -> (element=w195:string)
            n150 = property on="Levels" class="DigNum (strict)"("Visible"=w212) -> ()  [unwired: 2 in, 2 out]
            n151 = property on="Interval" class="DigNum (strict)"("Visible"=w211) -> ()  [unwired: 2 in, 2 out]
            n152 = property on="Level List" class="LstBox (strict)"("Visible"=w210) -> ()  [unwired: 2 in, 2 out]
            n153 = property on="Anchored at" class="Bool (strict)"("Visible"=w209) -> ()  [unwired: 2 in, 2 out]
            n154 = property on="Anchored Num" class="DigNum (strict)"("Visible"=w209) -> ()  [unwired: 2 in, 2 out]
            n155 = Decimal String To Number(string=w195) -> (number=w191:i32)  [unwired: 3 out]
            n156 = call <vilib>:"get_plot_property.vi"("Plot ID"=w191, "Plot Properties Array"=w194) -> ("index of element"=w190:i32, "element"=w193:T4)  [unwired: 1 in, 7 out]
            n157 = for {
              tunnel: w199 -> [w250] mode=indexing
              tunnel: [w249] -> w214 mode=indexing
              n158 = Fract/Exp String To Number(string=w250) -> (number=w249:dbl)  [unwired: 4 out]
            }
            n159 = Bundle By Name(cluster=w193, "Contour Properties.Contour color"="Contour Color", "Contour Properties.Axis"="Contour Direction", "Contour Properties.Draw contour"="Contour Draw", "Contour Properties.Antialias"="Contour Antialiasing", "Contour Properties.Line Width"="Contour Width", "Contour Properties.Levels"="Levels", "Contour Properties.Intervals"="Interval", "Contour Properties.Anchored"="Anchored at", "Contour Properties.Anchored At"="Anchored Num", "Contour Properties.Mode"="Mode", "Contour Properties.Contour Line Style"="Contour Line Style", "Contour Properties.Level List"=w214) -> (w221:T4)
            n160 = Replace Array Subset(array=w194, new element=w221, index=w190) -> (w220:T3)
          }
          event "Level List": Key Down {
            n161 = event-data() -> ("VKey"=w255:T13)  [unwired: 10 out]
            n162 = Equal?(x=w255, y=eventvkey."Delete" ("VKey")) -> (x = y?=w253:bool)
            n163 = case shown="True" w253 {
              tunnel: w252 -> [w256 w261]
              tunnel: [w256 w260] -> w251
              frame False {
              }
              frame True {
                n164 = local read "add new"() -> (w258:string)
                n165 = property on="Level List" class="LstBox (strict)"() -> ("Item Names"=w259:string[])  [unwired: 2 in, 2 out]
                n166 = local read "add new"() -> (w257:string)
                n167 = Index Array(array=w259, index="Level List") -> (element=w273:string)
                n168 = property on="Plots" class="LstBox (strict)"() -> ("Value"=w270:i32)  [unwired: 2 in, 2 out]
                n169 = Equal?(x=w273, y=w257) -> (x = y?=w272:bool)
                n170 = case shown="True" w272 {
                  tunnel: w259 -> [w284 w285]
                  tunnel: "Level List" -> [w283 _]
                  tunnel: [w282 w285] -> w262
                  frame False {
                    n171 = Delete From Array(array=w284, index=w283) -> (array with subset deleted=w282:string[])  [unwired: 1 in, 1 out]
                    n172 = property on="Level List" class="LstBox (strict)"("Item Names"=w282) -> ()  [unwired: 2 in, 2 out]
                  }
                  frame True {
                  }
                }
                n173 = Search 1D Array(1D array=w262, element=w258) -> (index of element=w265:i32)  [unwired: 1 out]
                n174 = Equal?(x=w265, y=-1) -> (x = y?=w264:bool)
                n175 = case shown="False" w264 {
                  tunnel: w262 -> [w274 w279]
                  tunnel: [w275 w279] -> w266
                  tunnel: w265 -> [w276 _]
                  frame False {
                    n176 = Delete From Array(array=w274, index=w276) -> (array with subset deleted=w275:string[])  [unwired: 1 in, 1 out]
                  }
                  frame True {
                    n177 = local read "add new"() -> (w277:string)
                    n178 = Insert Into Array(array=w279, new element=w277) -> (w278:string[])  [unwired: 1 in]
                    n179 = property on="Level List" class="LstBox (strict)"("Item Names"=w278) -> ()  [unwired: 2 in, 2 out]
                  }
                }
                n180 = Index Array(array=w261, index=w270) -> (element=w267:T4)
                n181 = for {
                  tunnel: w266 -> [w281] mode=indexing
                  tunnel: [w280] -> w268 mode=indexing
                  n182 = Fract/Exp String To Number(string=w281) -> (number=w280:dbl)  [unwired: 4 out]
                }
                n183 = Bundle By Name(cluster=w267, "Contour Properties.Level List"=w268) -> (w269:T4)
                n184 = Replace Array Subset(array=w261, new element=w269, index=w270) -> (w260:T3)
              }
            }
          }
          event "Normal Antialiasing", "Normal Draw", "Normal Width", "Normal Length", "Normal Color": Value Change {
            n185 = event-data() -> ()  [unwired: 7 out]
            n186 = property on="Plots" class="LstBox (strict)"() -> ("Value"=w290:i32)  [unwired: 2 in, 2 out]
            n187 = property on="Plots" class="LstBox (strict)"() -> ("Item Names"=w292:string[])  [unwired: 2 in, 2 out]
            n188 = Index Array(array=w292, index=w290) -> (element=w291:string)
            n189 = Decimal String To Number(string=w291) -> (number=w287:i32)  [unwired: 3 out]
            n190 = call <vilib>:"get_plot_property.vi"("Plot ID"=w287, "Plot Properties Array"=w289) -> ("index of element"=w286:i32, "element"=w288:T4)  [unwired: 1 in, 7 out]
            n191 = Bundle By Name(cluster=w288, "Normal Properties.Normal color"="Normal Color", "Normal Properties.Normal Length"="Normal Length", "Normal Properties.Normal Width"="Normal Width", "Normal Properties.Draw Normal"="Normal Draw", "Normal Properties.Antialiasing"="Normal Antialiasing") -> (w299:T4)
            n192 = Replace Array Subset(array=w289, new element=w299, index=w286) -> (w298:T3)
          }
          event "Plots": Value Change {
            n193 = event-data() -> ("OldVal"=w301:i32)  [unwired: 6 out]
            n194 = property on="Color Ramp" class="ColRmp (strict)"() -> ("Scale.MarkerVals[]"=w307:cluster{dbl, u32}[])  [unwired: 2 in, 2 out]
            n195 = property on="Plots" class="LstBox (strict)"() -> ("Item Names"=w305:string[])  [unwired: 2 in, 2 out]
            n196 = Index Array(array=w305, index=w301) -> (element=w304:string)
            n197 = Decimal String To Number(string=w304) -> (number=w306:i32)  [unwired: 3 out]
            n198 = call <vilib>:"get_plot_property.vi"("Plot ID"=w306, "Plot Properties Array"=w302) -> ("index of element"=w300:i32, "element"=w303:T4)  [unwired: 1 in, 7 out]
            n199 = Bundle By Name(cluster=w303, "Surface Properties.Color Map"=w307) -> (w309:T4)
            n200 = Replace Array Subset(array=w302, new element=w309, index=w300) -> (w308:T3)
          }
          event "Tab Plot Prop": Mouse Leave {
            n201 = event-data() -> ()  [unwired: 5 out]
            n202 = property on="Color Ramp" class="ColRmp (strict)"() -> ("Scale.MarkerVals[]"=w318:cluster{dbl, u32}[])  [unwired: 2 in, 2 out]
            n203 = property on="Plots" class="LstBox (strict)"() -> ("Value"=w314:i32)  [unwired: 2 in, 2 out]
            n204 = property on="Plots" class="LstBox (strict)"() -> ("Item Names"=w316:string[])  [unwired: 2 in, 2 out]
            n205 = Index Array(array=w316, index=w314) -> (element=w315:string)
            n206 = Decimal String To Number(string=w315) -> (number=w317:i32)  [unwired: 3 out]
            n207 = call <vilib>:"get_plot_property.vi"("Plot ID"=w317, "Plot Properties Array"=w312) -> ("index of element"=w311:i32, "element"=w313:T4)  [unwired: 1 in, 7 out]
            n208 = Bundle By Name(cluster=w313, "Surface Properties.Color Map"=w318) -> (w320:T4)
            n209 = Replace Array Subset(array=w312, new element=w320, index=w311) -> (w319:T3)
          }
          event User Event {
            n210 = event-data() -> ()  [unwired: 6 out]
            n211 = property on="Plots" class="LstBox (strict)"() -> ("Value"=w327:i32)  [unwired: 2 in, 2 out]
            n212 = property on="Color Ramp" class="ColRmp (strict)"() -> ("Scale.MarkerVals[]"=w331:cluster{dbl, u32}[], "Scale.Interpolate Color"=w321:bool)  [unwired: 2 in, 2 out]
            n213 = property on="Plots" class="LstBox (strict)"() -> ("Item Names"=w323:string[])  [unwired: 2 in, 2 out]
            n214 = Index Array(array=w323, index=w327) -> (element=w328:string)
            n215 = Decimal String To Number(string=w328) -> (number=w325:i32)  [unwired: 3 out]
            n216 = call <vilib>:"get_plot_property.vi"("Plot ID"=w325, "Plot Properties Array"=w322) -> ("index of element"=w324:i32, "element"=w326:T4)  [unwired: 1 in, 7 out]
            n217 = Bundle By Name(cluster=w326, "Surface Properties.Color Map"=w331, "Surface Properties.Interpolate Color"=w321) -> (w332:T4)
            n218 = flat-sequence {
              tunnel: w330 -> [w334]
              tunnel: [w334] -> w329
              frame #0 {
                n219 = control-ref of="This VI"() -> (w336:refnum<vi>)
                n220 = Generate User Event(user event="done", event data cluster=w336) -> ()  [unwired: 2 in, 2 out]
              }
            }
            n221 = Replace Array Subset(array=w322, new element=w332, index=w324) -> (w330:T3)
          }
          event "Add Plot": Value Change {
            n222 = event-data() -> ("NewVal"=w340:bool)  [unwired: 6 out]
            n223 = case shown="True" w340 {
              tunnel: w339 -> [w341 w352]
              tunnel: [w341 w351] -> w338
              frame False {
              }
              frame True {
                n224 = property on="Plots" class="LstBox (strict)"() -> ("Item Names"=w347:string[])  [unwired: 2 in, 2 out]
                n225 = Array Size(array=w347) -> (size(s)=w343:i32)
                n226 = Bundle By Name(cluster=T4 {"Projection Properties"={"Draw XY"=FALSE, "Draw YZ"=FALSE, "Draw XZ"=FALSE}, "Surface Properties"={"Draw surface"=FALSE, "Opacity"=0.0, "Shading"=FALSE, "Specular"=0, "Color Map"=[], "Interpolate Color"=TRUE, "Absolute Colormap"=FALSE}, "Contour Properties"={"Contour color"=0, "Axis"=enum."X", "Draw contour"=FALSE, "Antialias"=FALSE, "Line Width"=0.0, "Contour Line Style"=enum."Solid", "Mode"=enum."Levels", "Levels"=0.0, "Intervals"=0.0, "Anchored At"=0.0, "Anchored"=FALSE, "Level List"=[]}, "Normal Properties"={"Normal color"=0, "Normal Length"=0.0, "Normal Width"=0.0, "Draw Normal"=FALSE, "Antialiasing"=FALSE}, "Points/Lines Properties"={"Color"=0, "Antialiasing"=FALSE, "Point Size"=0.0, "Points / Lines"=enum."None", "Point Style"=enum."Point", "Line Style"=enum."Solid", "Line Width"=0.0}, "Plot ID"=0, "Coordinate System"=enum."Cartesian"} ("Plot Properties"), "Plot ID"=w343) -> (w342:T4)
                n227 = Number To Decimal String(number=w343) -> (decimal integer string=w350:string)  [unwired: 1 out]
                n228 = Build Array (concatenate)(w352, w342) -> (w351:T3)
                n229 = Greater?(x=w343, y=10) -> (0:w345:bool)
                n230 = Build Array (concatenate)(w347, w350) -> (w349:string[])
                n231 = case shown="True" w345 {
                  selector: w345 -> [w353 w354]
                  frame False {
                    n232 = property on="Plots" class="LstBox (strict)"("Scrollbar Visible"=w353) -> ()  [unwired: 2 in, 2 out]
                  }
                  frame True {
                    n233 = property on="Plots" class="LstBox (strict)"("Scrollbar Visible"=w354) -> ()  [unwired: 2 in, 2 out]
                  }
                }
                n234 = property on="Plots" class="LstBox (strict)"("Item Names"=w349) -> (error out=w348:errorcluster)  [unwired: 2 in, 1 out]
                n235 = property on="Plots" class="LstBox (strict)"(error in=w348, "Value"=w343) -> ()  [unwired: 1 in, 2 out]
              }
            }
          }
          event "Projection Draw XZ", "Projection Draw XY", "Projection Draw YZ": Value Change {
            n236 = event-data() -> ()  [unwired: 7 out]
            n237 = property on="Plots" class="LstBox (strict)"() -> ("Value"=w358:i32)  [unwired: 2 in, 2 out]
            n238 = property on="Plots" class="LstBox (strict)"() -> ("Item Names"=w360:string[])  [unwired: 2 in, 2 out]
            n239 = Index Array(array=w360, index=w358) -> (element=w359:string)
            n240 = Decimal String To Number(string=w359) -> (number=w361:i32)  [unwired: 3 out]
            n241 = call <vilib>:"get_plot_property.vi"("Plot ID"=w361, "Plot Properties Array"=w357) -> ("index of element"=w355:i32, "element"=w356:T4)  [unwired: 1 in, 7 out]
            n242 = Bundle By Name(cluster=w356, "Projection Properties.Draw XY"="Projection Draw XY", "Projection Properties.Draw YZ"="Projection Draw YZ", "Projection Properties.Draw XZ"="Projection Draw XZ") -> (w363:T4)
            n243 = Replace Array Subset(array=w357, new element=w363, index=w355) -> (w362:T3)
          }
          event "PL Antialiasing", "PL Color", "Point Size", "Points/Lines", "Point Style", "Line Style", "Line Width": Value Change {
            n244 = event-data() -> ()  [unwired: 7 out]
            n245 = property on="Plots" class="LstBox (strict)"() -> ("Value"=w370:i32)  [unwired: 2 in, 2 out]
            n246 = property on="Plots" class="LstBox (strict)"() -> ("Item Names"=w372:string[])  [unwired: 2 in, 2 out]
            n247 = Index Array(array=w372, index=w370) -> (element=w371:string)
            n248 = Decimal String To Number(string=w371) -> (number=w373:i32)  [unwired: 3 out]
            n249 = case shown="0, Default" "Points/Lines" {
              tunnel: [_ TRUE ("Visible") FALSE ("Visible") w395] -> w375
              tunnel: [_ FALSE ("Visible") TRUE ("Visible") w395] -> w374
              frame 0, Default {
              }
              frame 1 {
              }
              frame 2 {
                n250 = property on="Line Width" class="DigNum (strict)"("Position"=T12 {"Left"=-144, "Top"=-650} ("Position 3")) -> ()  [unwired: 2 in, 2 out]
                n251 = property on="Line Style" class="Ring (strict)"("Position"=T12 {"Left"=-243, "Top"=-649} ("Position 2")) -> ()  [unwired: 2 in, 2 out]
              }
              frame 3 {
                w395 = TRUE ("Visible")
                n252 = property on="Line Style" class="Ring (strict)"("Position"=T12 {"Left"=-243, "Top"=-609} ("Position 4")) -> ()  [unwired: 2 in, 2 out]
                n253 = property on="Point Style" class="Ring (strict)"("Position"=T12 {"Left"=-243, "Top"=-649} ("Position 2")) -> ()  [unwired: 2 in, 2 out]
                n254 = property on="Line Width" class="DigNum (strict)"("Position"=T12 {"Left"=-144, "Top"=-610} ("Position 5")) -> ()  [unwired: 2 in, 2 out]
                n255 = property on="Point Size" class="DigNum (strict)"("Position"=T12 {"Left"=-144, "Top"=-650} ("Position 3")) -> ()  [unwired: 2 in, 2 out]
              }
            }
            n256 = call <vilib>:"get_plot_property.vi"("Plot ID"=w373, "Plot Properties Array"=w368) -> ("index of element"=w367:i32, "element"=w369:T4)  [unwired: 1 in, 7 out]
            n257 = Bundle By Name(cluster=w369, "Points/Lines Properties.Color"="PL Color", "Points/Lines Properties.Points / Lines"="Points/Lines", "Normal Properties.Antialiasing"="PL Antialiasing", "Points/Lines Properties.Point Size"="Point Size", "Points/Lines Properties.Point Style"="Point Style", "Points/Lines Properties.Line Style"="Line Style", "Points/Lines Properties.Line Width"="Line Width") -> (w384:T4)
            n258 = property on="Line Width" class="DigNum (strict)"("Visible"=w374) -> ()  [unwired: 2 in, 2 out]
            n259 = property on="Point Style" class="Ring (strict)"("Visible"=w375) -> ()  [unwired: 2 in, 2 out]
            n260 = property on="Point Size" class="DigNum (strict)"("Visible"=w375) -> ()  [unwired: 2 in, 2 out]
            n261 = property on="Line Style" class="Ring (strict)"("Visible"=w374) -> ()  [unwired: 2 in, 2 out]
            n262 = Replace Array Subset(array=w368, new element=w384, index=w367) -> (w383:T3)
          }
          event "Surface Shading", "Surface Opacity", "Surface Draw", "Coordinate System", "Color Map Mode": Value Change; "Color Ramp": Shortcut Menu Selection (App) {
            n263 = event-data() -> ()  [unwired: 5 out]
            n264 = property on="Color Ramp" class="ColRmp (strict)"() -> ("Scale.MarkerVals[]"=w412:cluster{dbl, u32}[], "Scale.Interpolate Color"=w398:bool)  [unwired: 2 in, 2 out]
            n265 = In Range and Coerce(upper limit=1.0, x="Surface Opacity", lower limit=0.0) -> (coerced(x)=w406:dbl, In Range?=w408:bool)
            n266 = case shown="True" w408 {
              tunnel: w406 -> [w419 _]
              frame False {
                n267 = local write "Surface Opacity"(w419) -> ()
              }
              frame True {
              }
            }
            n268 = property on="Plots" class="LstBox (strict)"() -> ("Value"=w402:i32)  [unwired: 2 in, 2 out]
            n269 = case shown="1" "Color Map Mode" {
              tunnel: [TRUE ("Surface Properties.Absolute Colormap") FALSE ("Surface Properties.Absolute Colormap")] -> w396
              frame 0, Default {
              }
              frame 1 {
              }
            }
            n270 = property on="Plots" class="LstBox (strict)"() -> ("Item Names"=w404:string[])  [unwired: 2 in, 2 out]
            n271 = Index Array(array=w404, index=w402) -> (element=w403:string)
            n272 = Decimal String To Number(string=w403) -> (number=w405:i32)  [unwired: 3 out]
            n273 = call <vilib>:"get_plot_property.vi"("Plot ID"=w405, "Plot Properties Array"=w401) -> ("index of element"=w399:i32, "element"=w400:T4)  [unwired: 1 in, 7 out]
            n274 = Bundle By Name(cluster=w400, "Surface Properties.Draw surface"="Surface Draw", "Surface Properties.Color Map"=w412, "Surface Properties.Opacity"=w406, "Surface Properties.Shading"="Surface Shading", "Coordinate System"="Coordinate System", "Surface Properties.Interpolate Color"=w398, "Surface Properties.Absolute Colormap"=w396) -> (w416:T4)
            n275 = Replace Array Subset(array=w401, new element=w416, index=w399) -> (w415:T3)
          }
        }
        n276 = Enqueue Element(queue=w160, element=w158) -> (queue out=w159:refnum<queue>)  [unwired: 1 in, 3 out]
      }
    }
  }
  "Plot Properties Out" <- w9
  n277 = Release Queue(queue=w8) -> ()  [unwired: 1 in, 4 out]
